vi "forvard - filter.vi"(5 "intensity/phase":i16(ring) items=["int", "pha"], 6 "path filter in":string, 7 "multiplication/substitution":i16(ring) items=["subst", "mult"], 8 "forward distance":dbl, 10 "field":T1) -> (1 "forwarded dist":dbl=1.0, 2 "Path Filter":string, 3 "field out":T1)   [LabVIEW 2012, in "LightPipes.lvlib"]
uses:
  LightPipes.lvlib
panel:
  # "FILTER"
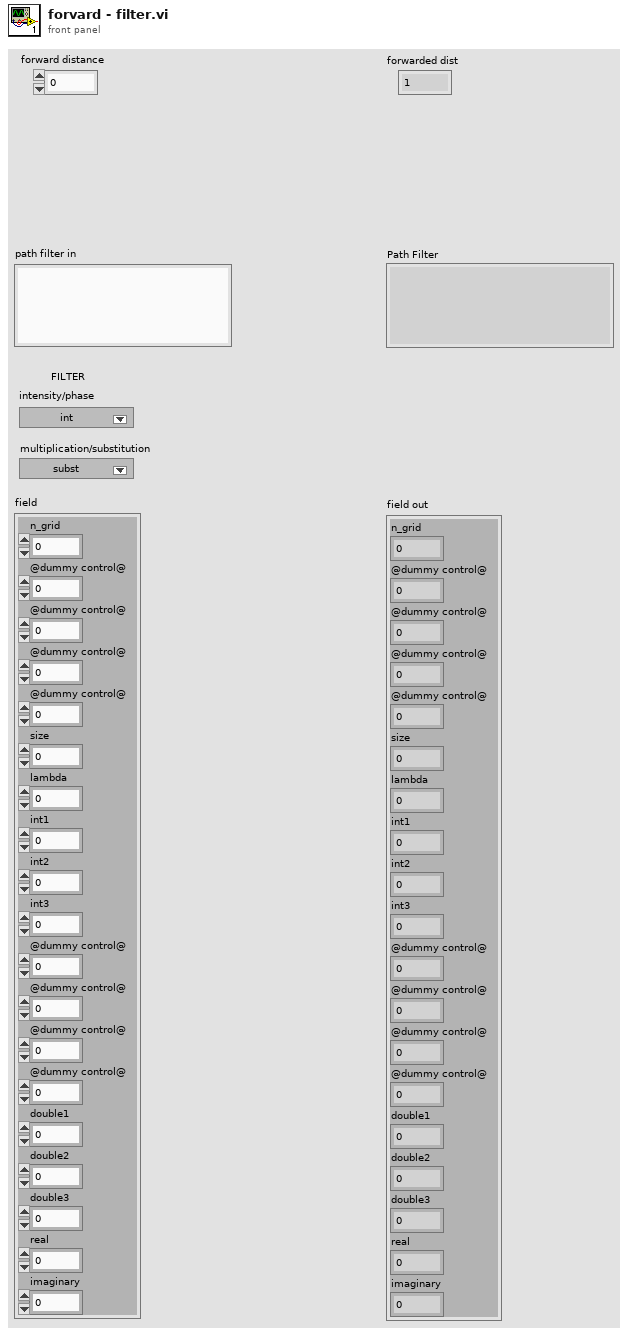
[diagram p1: front panel]
types:
  T1 = cluster{"n_grid":i32, "@dummy control@":i8, "@dummy control@":i8, "@dummy control@":i8, "@dummy control@":i8, "size":dbl, "lambda":dbl, "int1":i32, "int2":i32, "int3":i32, "@dummy control@":i8, "@dummy control@":i8, "@dummy control@":i8, "@dummy control@":i8, "double1":dbl, "double2":dbl, "double3":dbl, "real":u32, "imaginary":u32}
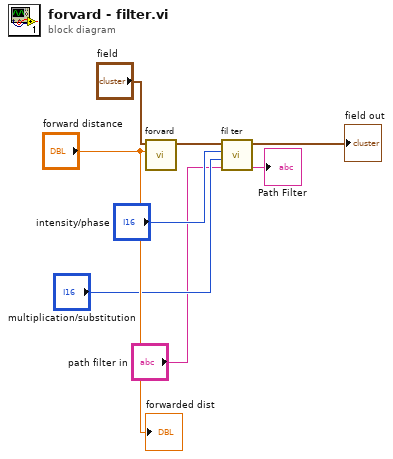
[diagram p0: block diagram]
diagram:
  n1 = call "forvard.vi"("distance"="forward distance", "field"="field") -> ("field out"=w3:T1)  [unwired: 9 in]
  n2 = call "fil ter.vi"("Path"="path filter in", "multiplication/ substitution"="multiplication/substitution", "intensity / phase"="intensity/phase", "field"=w3) -> ("Path Filter"=→"Path Filter":string, "field out"=→"field out":T1)  [unwired: 6 in]
  "forwarded dist" <- "forward distance"
